vi "Fifo (SubVI).vi"(4 "duration":dbl, 6 "y":dbl, 7 "Actual Sample Rate (dt)":dbl, 9 "Rotation [RPS]":dbl, 10 "Measurement in":waveform(dbl)[](array[waveform]), 11 "appended array":waveform(dbl)[](array[waveform])) -> (3 "Array":waveform(dbl)[](array[waveform]))   [LabVIEW 2012]
uses:
  <vilib>/Waveform/WDTOps.llb/WDT Append Waveforms DBL.vi
  <vilib>/Waveform/WDTOps.llb/WDT Waveform Duration DBL.vi
  <vilib>/Waveform/WDTOps.llb/WDT Get Waveform Subset DBL.vi
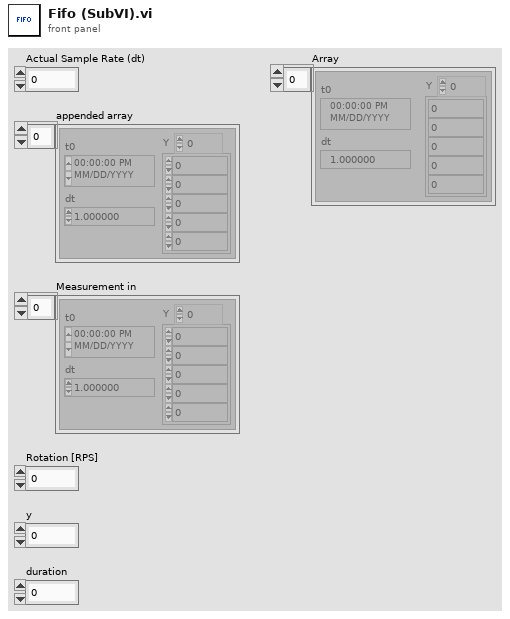
[diagram p1: front panel]
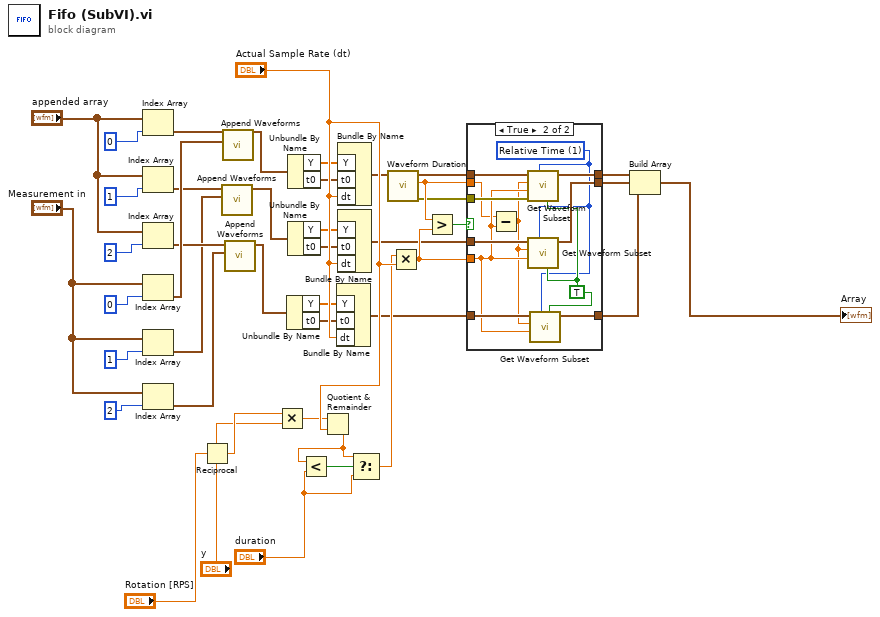
[diagram p0: block diagram]
diagram:
  n1 = Index Array(array="appended array", index=0 ("disabled index (col)")) -> (element=w9:waveform(dbl))
  n2 = Index Array(array="appended array", index=1 ("disabled index (col)")) -> (element=w10:waveform(dbl))
  n3 = Index Array(array="appended array", index=2 ("disabled index (col)")) -> (element=w11:waveform(dbl))
  n4 = Index Array(array="Measurement in", index=0 ("disabled index (col)")) -> (element=w14:waveform(dbl))
  n5 = Index Array(array="Measurement in", index=1 ("disabled index (col)")) -> (element=w8:waveform(dbl))
  n6 = Index Array(array="Measurement in", index=2 ("disabled index (col)")) -> (element=w7:waveform(dbl))
  n7 = Reciprocal(x="Rotation [RPS]") -> (1/x=w36:dbl)
  n8 = call-poly <vilib>:"Append Waveforms.vi"("waveform B"=w8, "waveform A"=w10) -> ("waveform out"=w22:waveform(dbl))  [unwired: 8 in, 1 out]
  n9 = call-poly <vilib>:"Append Waveforms.vi"("waveform B"=w14, "waveform A"=w9) -> ("waveform out"=w21:waveform(dbl))  [unwired: 8 in, 1 out]
  n10 = call-poly <vilib>:"Append Waveforms.vi"("waveform B"=w7, "waveform A"=w11) -> ("waveform out"=w23:waveform(dbl))  [unwired: 8 in, 1 out]
  n11 = Multiply(x=w36, y="y") -> (x*y=w37:dbl)
  n12 = Unbundle By Name(w23) -> ("Y"=w20:dbl[], "t0"=w19:timestamp)
  n13 = Unbundle By Name(w21) -> ("Y"=w16:dbl[], "t0"=w15:timestamp)
  n14 = Unbundle By Name(w22) -> ("Y"=w17:dbl[], "t0"=w18:timestamp)
  n15 = Quotient & Remainder(x=w37, y="Actual Sample Rate (dt)") -> (floor(x/y)=w38:dbl)  [unwired: 1 out]
  n16 = Less?(x=w38, y="duration") -> (x < y?=w43:bool)
  n17 = Bundle By Name("Y"=w20, "t0"=w19, "dt"="Actual Sample Rate (dt)") -> (w29:waveform(dbl))  [unwired: 1 in]
  n18 = Bundle By Name("Y"=w16, "t0"=w15, "dt"="Actual Sample Rate (dt)") -> (w25:waveform(dbl))  [unwired: 1 in]
  n19 = Bundle By Name("Y"=w17, "t0"=w18, "dt"="Actual Sample Rate (dt)") -> (w28:waveform(dbl))  [unwired: 1 in]
  n20 = Select(t=w38, s=w43, f="duration") -> (s? t:f=w35:dbl)
  n21 = call-poly <vilib>:"Waveform Duration.vi"("waveform in"=w25) -> ("error out"=w24:errorcluster, "duration"=w30:dbl, "waveform out"=w27:waveform(dbl))  [unwired: 8 in]
  n22 = Multiply(x=w35, y="Actual Sample Rate (dt)") -> (x*y=w31:dbl)
  n23 = Greater?(x=w30, y=w31) -> (0:w32:bool)
  n24 = case shown="True" w32 {
    tunnel: w24 -> [_ w59]
    tunnel: [w47 w58] -> w26
    tunnel: w27 -> [w47 w57]
    tunnel: w28 -> [w46 w56]
    tunnel: [w46 w55] -> w41
    tunnel: w29 -> [w45 w54]
    tunnel: w31 -> [_ w52]
    tunnel: w30 -> [_ w50]
    tunnel: [w45 w48] -> w42
    frame False {
    }
    frame True {
      w53 = TRUE ("open interval? (T)")
      w49 = u16 1 items=["Samples", "Relative Time"] ("start/duration format")
      n25 = Subtract(x=w50, y=w52) -> (x-y=w51:dbl)
      n26 = call-poly <vilib>:"Get Waveform Subset.vi"("open interval? (T)"=w53, "start/duration format"=w49, "error in (no error)"=w59, "duration"=w52, "start samples/time"=w51, "waveform in"=w57) -> ("waveform out"=w58:waveform(dbl))  [unwired: 3 out]
      n27 = call-poly <vilib>:"Get Waveform Subset.vi"("open interval? (T)"=w53, "start/duration format"=w49, "duration"=w52, "start samples/time"=w51, "waveform in"=w56) -> ("waveform out"=w55:waveform(dbl))  [unwired: 1 in, 3 out]
      n28 = call-poly <vilib>:"Get Waveform Subset.vi"("open interval? (T)"=w53, "start/duration format"=w49, "duration"=w52, "start samples/time"=w51, "waveform in"=w54) -> ("waveform out"=w48:waveform(dbl))  [unwired: 1 in, 3 out]
    }
  }
  n29 = Build Array(w26, w41, w42) -> (→"Array":waveform(dbl)[])
